vi "temp_gets.vi"   [LabVIEW 2013]
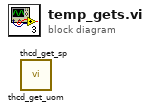
[diagram p0: block diagram]
diagram:
  n1 = call "thcd_get_uom.vi"() -> ()  [unwired: 6 in, 6 out]
  n2 = call "thcd_get_sp.vi"() -> ()  [unwired: 6 in, 6 out]
